vi "Disconnect UDB.vi"(8 "error in (no error)":errorcluster, 11 "Semiconductor Module Context":T1) -> (0 "error out":errorcluster)   [LabVIEW 2019]
uses:
  <vilib>/NI_TestStand_SemiconductorModule/NI_TestStand_Semiconductor_Module.lvlibp/PinMap/General/SemiconductorModuleContext.ctl
  <vilib>/DAQmx/write.llb/DAQmx Write (Digital 2D Bool NChan 1Samp NLine).vi
  <vilib>/DAQmx/read.llb/DAQmx Read (Digital U32 1Chan 1Samp).vi
  <vilib>/DAQmx/write.llb/DAQmx Write (Digital U32 1Chan 1Samp).vi
  <vilib>/DAQmx/miscellaneous.llb/DAQmx Fill In Error Info.vi
  <vilib>/NI_TestStand_SemiconductorModule/NI_TestStand_Semiconductor_Module.lvlibp
  <vilib>/DAQmx/write.llb/DAQmx Write (Digital 1D Bool 1Chan 1Samp).vi
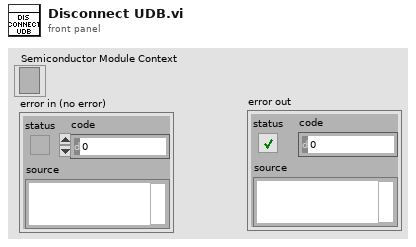
[diagram p1: front panel]
types:
  T1 = typedef "NI_TestStand_Semiconductor_Module.lvlibp/SemiconductorModuleContext.ctl" = refnum<k7>
  T2 = typedef "TSM DAQmx Multi-Task.ctl" = cluster{"Pin Query Context":refnum<class "MultiplePinMultipleSessionQueryContext.lvclass">, "SSC":T3[], "Site Numbers":i32[]}
  T3 = typedef "SSC DAQmx.ctl" = cluster{"DAQmx Task ":refnum<k21>, "Channels":string, "Channel Lists":string}
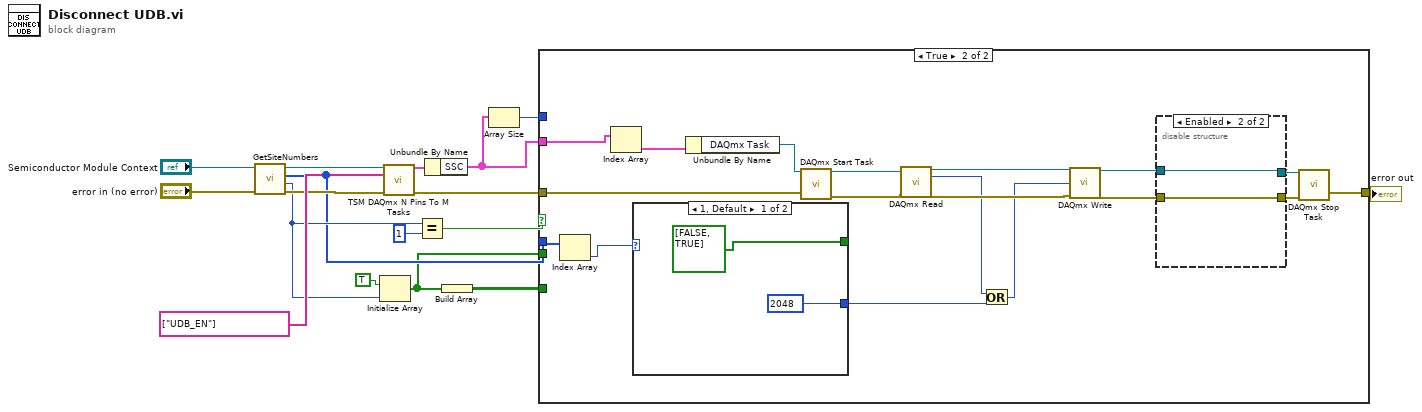
[diagram p0: block diagram]
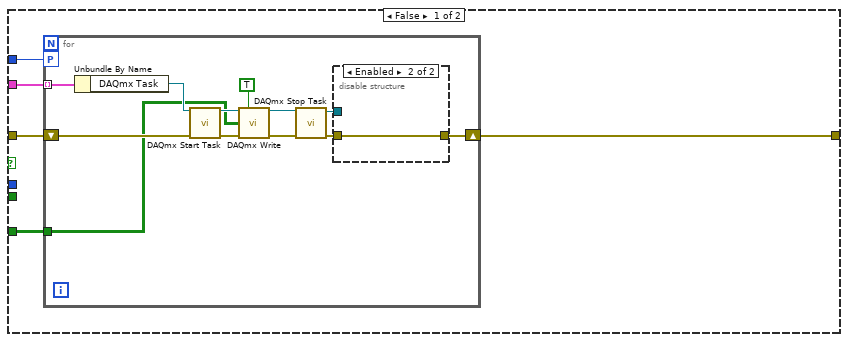
[diagram p2: hidden frame]
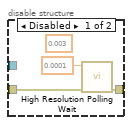
[diagram p3: hidden frame]
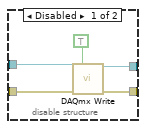
[diagram p4: hidden frame]
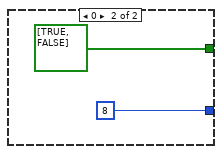
[diagram p5: hidden frame]
diagram:
  n1 = call <vilib>:"GetSiteNumbers.vi"("error in (no error)"="error in (no error)", "Semiconductor Module Context"="Semiconductor Module Context") -> ("error out"=w12:errorcluster, "Number Of Sites"=w5:i32, "Site Numbers"=w3:i32[], "Semiconductor Module Context Out"=w11:T1)  [unwired: 6 in]
  n2 = Initialize Array(TRUE ("element"), w5) -> (w2:bool[])
  n3 = call "TSM DAQmx N Pins To M Tasks.vi"("TSM context"=w11, "Pins"=tag[] ["UDB_EN"], "Site Numbers"=w3, "error in"=w12) -> ("DAQ TSM Out"=w13:T2, "error out"=w17:errorcluster)  [unwired: 10 in]
  n4 = Equal?(x=w5, y=1) -> (x = y?=w4:bool)
  n5 = Unbundle By Name(w13) -> ("SSC"=w14:T3[])
  n6 = Build Array(w2) -> (w7:bool[][])
  n7 = Array Size(array=w14) -> (size(s)=w15:i32)
  n8 = case shown="True" w4 {
    tunnel: w17 -> [w22 w53]
    tunnel: w15 -> [w21 _]
    tunnel: w14 -> [w20 w51]
    tunnel: w7 -> [w19 _]
    tunnel: [w18 w52] -> w6
    tunnel: w3 -> [_ w49]
    tunnel: w2 -> [_ _]
    frame False {
      n9 = for {
        shift-right: [w34] -> w18
        shift-left: w22 -> [w32]
        tunnel: w20 -> [w33] mode=indexing
        workers-P: w21 -> [_]
        tunnel: w19 -> [w23]
        n10 = Unbundle By Name(w33) -> ("DAQmx Task"=w24:refnum<k21>)
        n11 = call <vilib>:"DAQmx Start Task.vi"("task/channels in"=w24, "error in"=w32) -> ("task out"=w29:refnum<k21>, "error out"=w30:errorcluster)  [unwired: 12 in]
        n12 = call-poly <vilib>:"DAQmx Write.vi"("task/channels in"=w29, "auto start"=TRUE, "data"=w23, "error in"=w30) -> ("task out"=w28:refnum<k21>, "error out"=w27:errorcluster)  [unwired: 9 in, 1 out]
        n13 = call <vilib>:"DAQmx Stop Task.vi"("task/channels in"=w28, "error in"=w27) -> ("task out"=w25:refnum<k21>, "error out"=w26:errorcluster)  [unwired: 12 in]
        n14 = disable-structure shown="Enabled" {
          disable-tunnel: [w36 w38] -> w34
          disable-tunnel: w26 -> [w35 w38]
          disable-tunnel: w25 -> [_ _]
          frame Disabled {
            (unwired) 0.003 ("seconds to wait")
            n15 = call <vilib>:"High Resolution Polling Wait.vi"("error in (no error)"=w35, "seconds to wait"=0.0001) -> ("error out"=w36:errorcluster)  [unwired: 9 in]
          }
          frame Enabled {
          }
        }
      }
    }
    frame True {
      n16 = Index Array(array=w49) -> (element=w48:i32)  [unwired: 1 in]
      n17 = Index Array(array=w51) -> (element=w50:T3)  [unwired: 1 in]
      n18 = case shown="1, Default" w48 {
        tunnel: [bool[] [FALSE, TRUE] ("data") bool[] [TRUE, FALSE] ("data")] -> _
        tunnel: [u32 2048 u32 8] -> w40
        frame 1, Default {
        }
        frame 0 {
        }
      }
      n19 = Unbundle By Name(w50) -> ("DAQmx Task"=w54:refnum<k21>)
      n20 = call <vilib>:"DAQmx Start Task.vi"("task/channels in"=w54, "error in"=w53) -> ("task out"=w46:refnum<k21>, "error out"=w47:errorcluster)  [unwired: 12 in]
      n21 = call-poly <vilib>:"DAQmx Read.vi"("task/channels in"=w46, "error in"=w47) -> ("task out"=w43:refnum<k21>, "data"=w41:u32, "error out"=w45:errorcluster)  [unwired: 11 in]
      n22 = Or(x=w41, y=w40) -> (x .or. y?=w39:u32)
      n23 = call-poly <vilib>:"DAQmx Write.vi"("task/channels in"=w43, "data"=w39, "error in"=w45) -> ("task out"=w42:refnum<k21>, "error out"=w44:errorcluster)  [unwired: 10 in, 1 out]
      n24 = disable-structure shown="Enabled" {
        disable-tunnel: [w60 w62] -> w56
        disable-tunnel: [w59 w63] -> w55
        disable-tunnel: w44 -> [w58 w63]
        disable-tunnel: w42 -> [w57 w62]
        frame Disabled {
          n25 = call-poly <vilib>:"DAQmx Write.vi"("task/channels in"=w57, "auto start"=TRUE, "error in"=w58) -> ("task out"=w60:refnum<k21>, "error out"=w59:errorcluster)  [unwired: 10 in, 1 out]
        }
        frame Enabled {
        }
      }
      n26 = call <vilib>:"DAQmx Stop Task.vi"("task/channels in"=w56, "error in"=w55) -> ("error out"=w52:errorcluster)  [unwired: 12 in, 1 out]
    }
  }
  "error out" <- w6
